vi "Concatenar atualização de configurações para Log.vi"(1 "Seção/Key encontrada":bool, 2 "Leitura/Escrita":enum16{"Ler", "Gravar"}(ring), 3 "Key ja existia?":bool, 4 "Valor":string, 5 "Nome da Chave":string, 6 "Nome da Seção":string) -> (0 "Texto Concatenado":string)   [LabVIEW 2020]
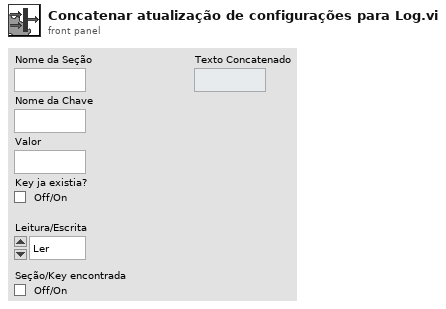
[diagram p1: front panel]
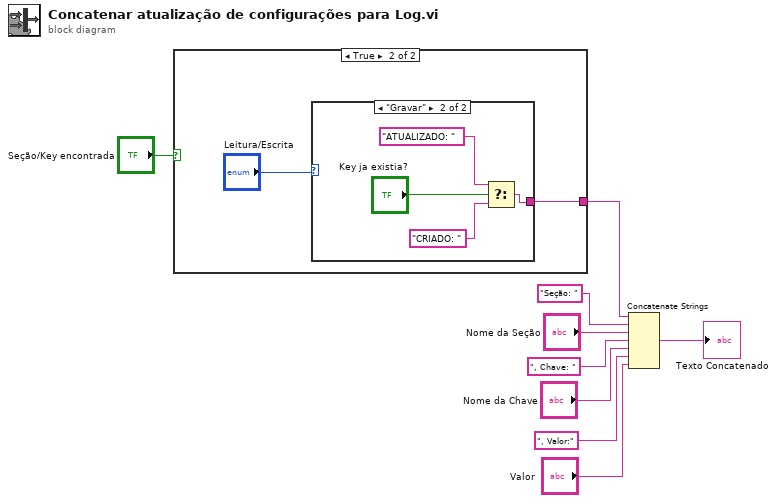
[diagram p0: block diagram]
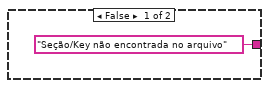
[diagram p2: hidden frame]
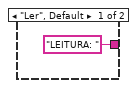
[diagram p3: hidden frame]
diagram:
  n1 = case shown="True" "Seção/Key encontrada" {
    tunnel: ["Seção/Key não encontrada no arquivo" w12] -> w9
    frame False {
    }
    frame True {
      n2 = case shown="\"Gravar\"" "Leitura/Escrita" {
        tunnel: ["LEITURA: " w17] -> w12
        frame "Ler", Default {
        }
        frame "Gravar" {
          n3 = Select(t="ATUALIZADO: ", s="Key ja existia?", f="CRIADO: ") -> (s? t:f=w17:string)
        }
      }
    }
  }
  n4 = Concatenate Strings(w9, "Seção: " ("string"), "Nome da Seção", ", Chave: " ("string"), "Nome da Chave", ", Valor:" ("string"), "Valor") -> (→"Texto Concatenado":string)
